vi "makeDecisions.vi"(8 "error in (no error)":errorcluster, 10 "model":refnum<class "Model.lvclass">, 11 "MovingToNewForceState in":refnum<class "SettlingState.lvclass">) -> (0 "error out":errorcluster, 2 "model 2":refnum<class "Model.lvclass">, 3 "MovingToNewForceState out":refnum<class "SettlingState.lvclass">)   [LabVIEW 2013, in "SettlingState.lvclass"]
uses:
  SettlingState.lvclass
  Model/Model/Model.lvclass
  MovingToNewTemperatureState/MovingToNewTemperatureState.lvclass
  Typedefs/StateSelector.ctl
  Typedefs/AITDTTypedefs.lvlib
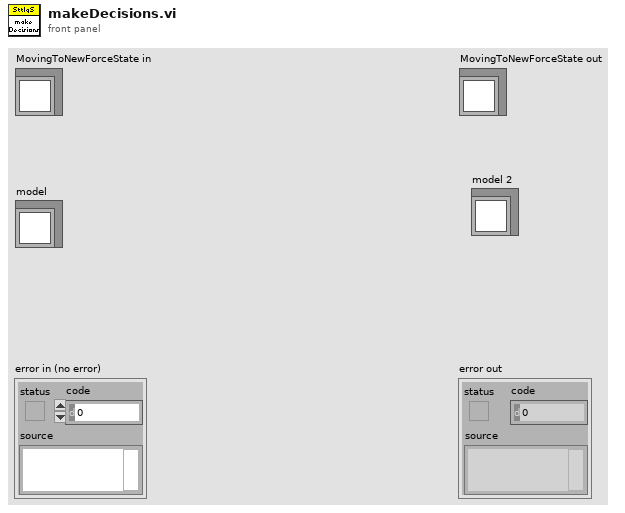
[diagram p1: front panel]
types:
  T1 = typedef "AITDTTypedefs.lvlib/StateSelector.ctl" = enum16{"AwaitingSetpointAcknowledgmentState", "EndingCycleState", "FaultState", "OffState", "PausingState", "RequestingNewSetpointState", "SamplingState", "SettlingState", "SoakingState", "StabilizingState", "StandbyState", "StoppedState", "TransitioningTemperatureState"}
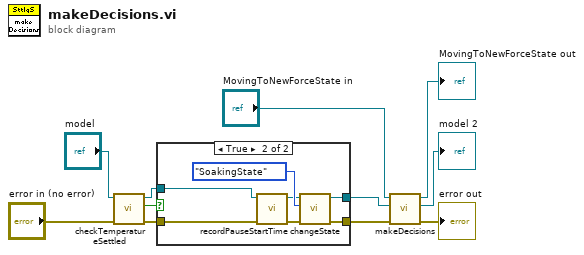
[diagram p0: block diagram]
diagram:
  n1 = call "checkTemperatureSettled.vi"("error in (no error)"="error in (no error)", "Model in"="model") -> ("error out"=w2:errorcluster, "tempSettledIsTrue"=w5:bool, "Model out"=w4:refnum<class "Model.lvclass">)  [unwired: 7 in]
  n2 = case shown="True" w5 {
    tunnel: w4 -> [w13 w19]
    tunnel: [w13 w17] -> w3
    tunnel: w2 -> [w12 w16]
    tunnel: [w12 w14] -> w1
    frame False {
    }
    frame True {
      n3 = call "recordPauseStartTime.vi"("error in (no error)"=w16, "Model in"=w19) -> ("error out"=w15:errorcluster, "Model out"=w18:refnum<class "Model.lvclass">)  [unwired: 8 in]
      n4 = call "changeState.vi"("error in (no error)"=w15, "State:"=StateSelector."SoakingState", "Model in"=w18) -> ("error out"=w14:errorcluster, "Model out"=w17:refnum<class "Model.lvclass">)  [unwired: 7 in]
    }
  }
  n5 = call-parent "makeDecisions.vi"("error in (no error)"=w1, "model"=w3, "EnabledState in"="MovingToNewForceState in") -> ("error out"=→"error out":errorcluster, "model 2"=→"model 2":refnum<class "Model.lvclass">, "EnabledState out"=→"MovingToNewForceState out":refnum<class "SettlingState.lvclass">)  [unwired: 6 in]
